vi "Replace Objects with DVRs.vi"(8 "error in (no error)":errorcluster, 10 "Class DVR Control File Path":path=path "D:/GitHub/LabVIEW/SLL/Tools/Class DVR API Generator/Example/My Sample Class.lvclass", 11 "DVR API Path":path=path "D:/GitHub/LabVIEW/SLL/Tools/Class DVR API Generator/Example/APIs/Sample Class Method API.vi") -> (0 "error out":errorcluster, 3 "DVR API Path Out":path=path "D:/GitHub/LabVIEW/SLL/Tools/Class DVR API Generator/Example/APIs/Sample Class Method API.vi")   [LabVIEW 2016, in "SLL Class DVR API Generator.lvlib"]
uses:
  SLL Class DVR API Generator.lvlib
  <vilib>/Utility/traverseref.llb/TRef TravTarget.ctl
  <vilib>/Utility/traverseref.llb/VI Scripting - Traverse.lvlib
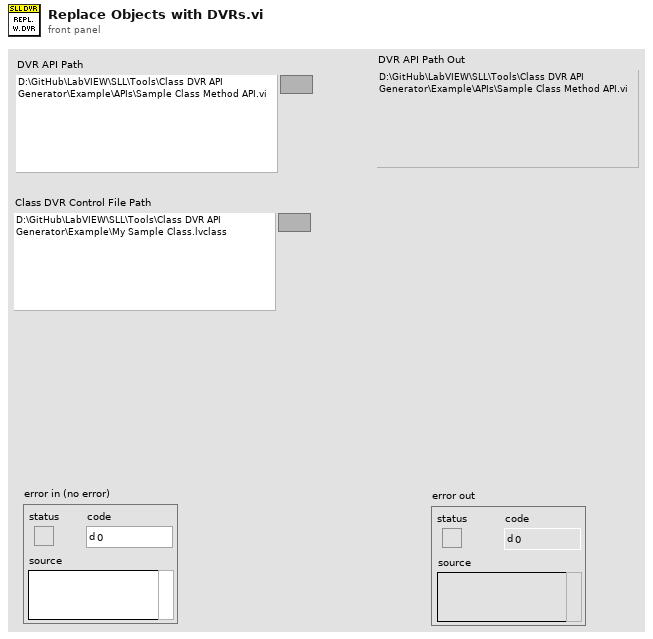
[diagram p1: front panel]
types:
  T1 = typedef "TRef TravTarget.ctl" = enum16{"FP", "BD", "Other"}
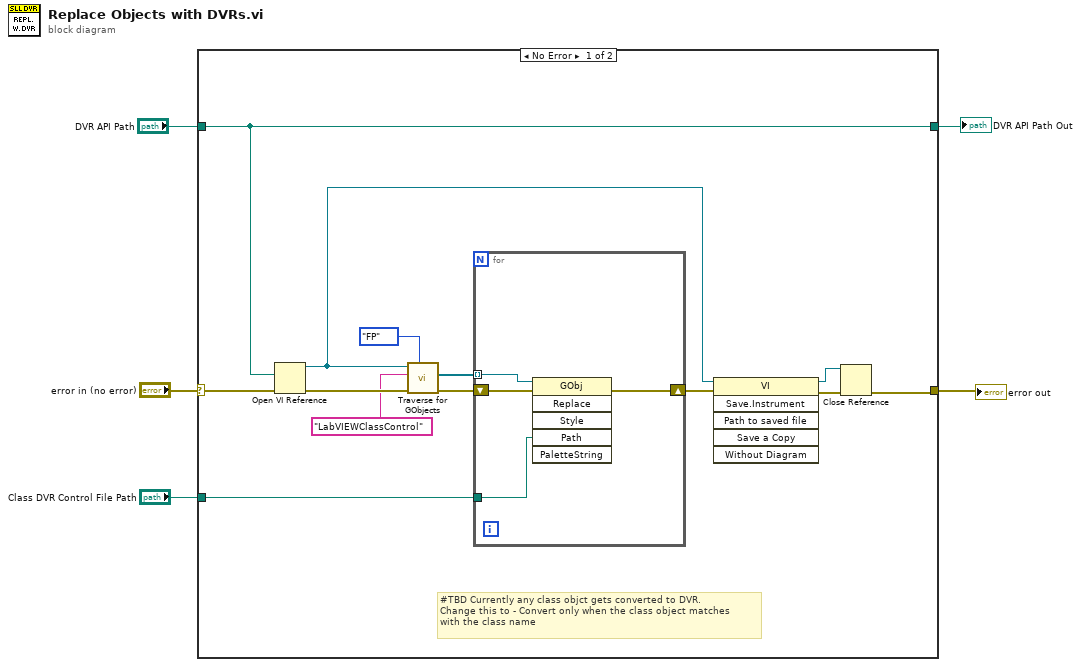
[diagram p0: block diagram]
diagram:
  n1 = case shown="No Error" "error in (no error)" {
    selector: "error in (no error)" -> [w18 w24]
    tunnel: [w7 w24] -> w4
    tunnel: "DVR API Path" -> [w6 w23]
    tunnel: "Class DVR Control File Path" -> [w12 _]
    tunnel: [w6 w23] -> w1
    frame No Error {
      # "#TBD Currently any class objct gets converted to DVR.\nChange this to - Convert only when the class object matches\nwith the class name"
      n2 = Open VI Reference(vi path=w6, error in (no error)=w18) -> (vi reference=w10:refnum<vi>, error out=w17:errorcluster)  [unwired: 4 in]
      n3 = call <vilib>:"Traverse for GObjects.vi"("Traverse Target"=TRef_TravTarget."FP", "error in (no error)"=w17, "Class Name"="LabVIEWClassControl", "VI Refnum"=w10) -> ("error out"=w13:errorcluster, "References"=w14:refnum<vi>[])  [unwired: 4 in, 2 out]
      n4 = for {
        tunnel: w14 -> [w21] mode=indexing
        tunnel: w12 -> [w20]
        shift-right: [w19] -> w11
        shift-left: w13 -> [w22]
        n5 = invoke class="GObj" method="Replace"(reference=w21, error in=w22, "Path"=w20) -> (error out=w19:errorcluster)  [unwired: 3 in, 5 out]
      }
      n6 = invoke class="VI" method="Save.Instrument"(reference=w10, error in=w11) -> (reference out=w8:refnum<vi>, error out=w9:errorcluster)  [unwired: 4 in, 4 out]
      n7 = Close Reference(reference=w8, error in (no error)=w9) -> (error out=w7:errorcluster)
    }
    frame Error {
    }
  }
  "error out" <- w4
  "DVR API Path Out" <- w1
